vi "Mod - Top VI.vi"(8 "error in":errorcluster) -> (0 "error out":errorcluster)   [LabVIEW 2024]
uses:
  Mod Queue - Dequeue.vi
  Mod Queue - Enqueue.vi
  Mod Queue - Destroy.vi
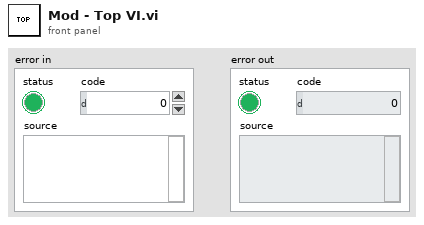
[diagram p1: front panel]
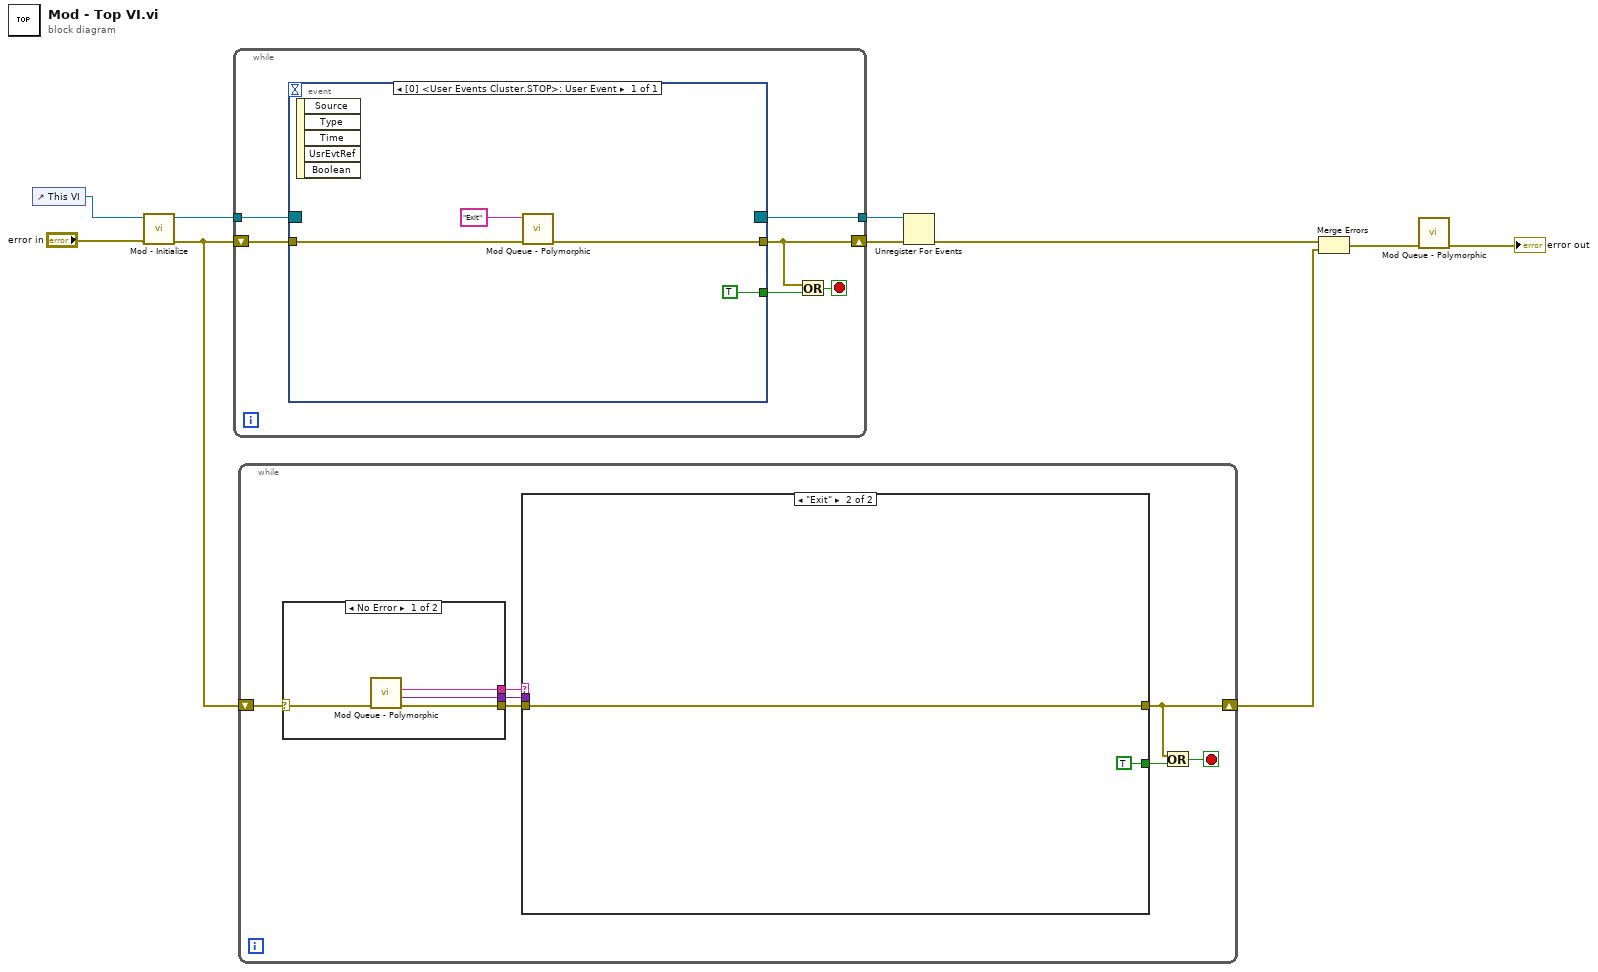
[diagram p0: block diagram]
diagram:
  n1 = control-ref of="This VI"() -> (w10:refnum<vi>)
  n2 = call "Mod - Initialize.vi"("error in (no error)"="error in", "VI In"=w10) -> ("error out"=w5:errorcluster, "Event Registration Out"=w8:refnum<event-registration>)  [unwired: 8 in]
  n3 = while {
    tunnel: w8 -> [w16]
    shift-right: [w11] -> w7
    shift-left: w5 -> [w15]
    tunnel: [w14] -> w6
    stop <- w12 stop-if-true
    n4 = event shown="[0] <User Events Cluster.STOP>: User Event" {
      selector: w16 -> [_]
      dyn-events: [_] -> w14
      timeout: _ -> [_]
      tunnel: w15 -> [w20]
      tunnel: [w19] -> w11
      tunnel: [TRUE] -> w13
      event User Event {
        n5 = event-data() -> ()  [unwired: 1 in, 5 out]
        n6 = call-poly "Mod Queue - Polymorphic.vi"("error in"=w20, "Message"="Exit") -> ("error out"=w19:errorcluster)  [unwired: 9 in]
      }
    }
    n7 = Or(x=w11, y=w13) -> (x .or. y?=w12:bool)
  }
  n8 = while {
    shift-right: [w21] -> w3
    shift-left: w5 -> [w27]
    stop <- w22 stop-if-true
    n9 = case shown="No Error" w27 {
      selector: w27 -> [w31 w35]
      tunnel: [w32 w35] -> w24
      tunnel: [w34 _] -> w26
      tunnel: [w33 _] -> w25
      frame No Error {
        n10 = call-poly "Mod Queue - Polymorphic.vi"("error in"=w31) -> ("error out"=w32:errorcluster, "Message Data"=w33:variant, "Message"=w34:string)  [unwired: 8 in]
      }
      frame Error {
      }
    }
    n11 = case shown="\"Exit\"" w26 {
      tunnel: w25 -> [_ _]
      tunnel: w24 -> [w28 w29]
      tunnel: [w28 w29] -> w21
      tunnel: [_ TRUE] -> w23
      frame "IDLE", Default {
      }
      frame "Exit" {
      }
    }
    n12 = Or(x=w21, y=w23) -> (x .or. y?=w22:bool)
  }
  n13 = Unregister For Events(event registration refnum=w6, error in=w7) -> (error out=w4:errorcluster)
  n14 = Merge Errors(w4, w3) -> (w2:errorcluster)
  n15 = call-poly "Mod Queue - Polymorphic.vi"("error in"=w2) -> ("error out"=→"error out":errorcluster)  [unwired: 10 in]
